vi "set_N_Dop.vi"(0 "Active":bool, 1 "Bubbler In":bool, 2 "H2 Dilute":bool, 3 "Gas Source In":bool, 4 "Run":bool, 5 "Remote":bool, 6 "Gas Flow":dbl, 8 "Flow 3":dbl, 10 "Flow 2":dbl, 12 "Flow 1":dbl) -> ()   [LabVIEW 2011]
uses:
  low_level_proc/globals.vi
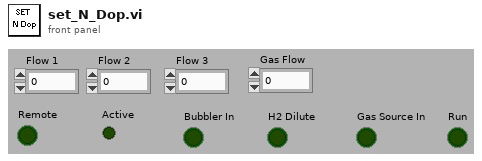
[diagram p1: front panel]
types:
  T1 = typedef "relaySpec.ctl" = cluster{"Card Index":u16, "Relay Index":u16}
  T2 = typedef "DA_Spec.ctl" = cluster{"Card Index":u16, "Channel Index":u16}
  T3 = cluster{"Relay Functions":cluster{"Remote":T1, "Active":T1, "Bubbler In":T1, "H2 dilute":T1, "Gas in":T1, "Run 2":T1}, "D/A Functions":cluster{"Flow 1":T2, "Flow 2":T2, "Flow 3":T2}, "Flow Ranges":cluster{"Flow 1 (NDOPMFC1)":u16, "Flow 2 (NDOPMFC2)":u16, "Flow 3 (NDOPMFC3)":u16, "Gas flow (NDOPMFC4)":u16}}
  T4 = cluster{"Remote":T1, "Active":T1, "Bubbler In":T1, "H2 dilute":T1, "Gas in":T1, "Run 2":T1}
  T5 = cluster{"Flow 1 (NDOPMFC1)":u16, "Flow 2 (NDOPMFC2)":u16, "Flow 3 (NDOPMFC3)":u16, "Gas flow (NDOPMFC4)":u16}
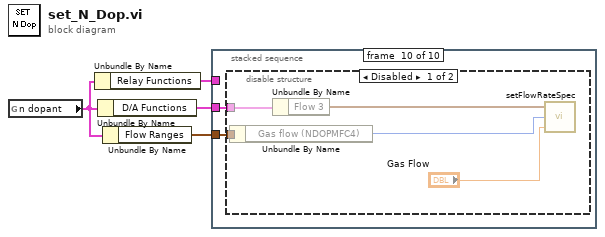
[diagram p0: block diagram]
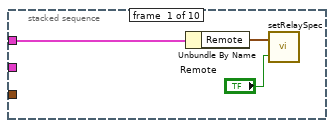
[diagram p2: hidden frame]
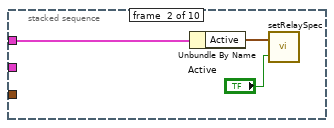
[diagram p3: hidden frame]
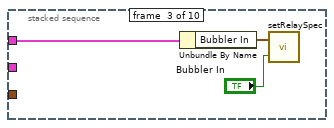
[diagram p4: hidden frame]
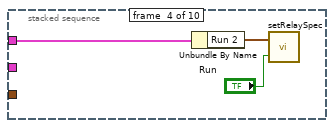
[diagram p5: hidden frame]
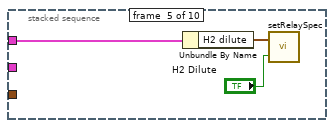
[diagram p6: hidden frame]
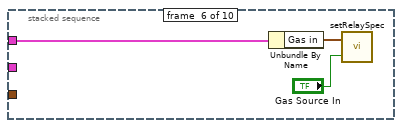
[diagram p7: hidden frame]
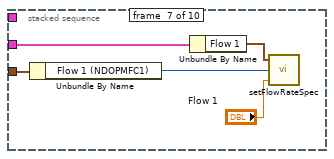
[diagram p8: hidden frame]
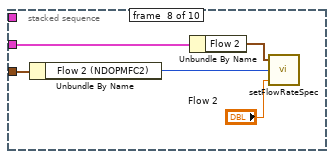
[diagram p9: hidden frame]
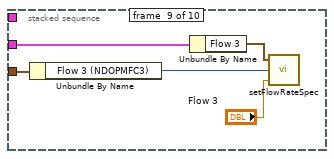
[diagram p10: hidden frame]
diagram:
  n1 = global read "globals.vi" "n dopant"() -> (w2:T3)
  n2 = Unbundle By Name(w2) -> ("Relay Functions"=w4:T4)
  n3 = Unbundle By Name(w2) -> ("D/A Functions"=w3:cluster{"Flow 1":T2, "Flow 2":T2, "Flow 3":T2})
  n4 = Unbundle By Name(w2) -> ("Flow Ranges"=w1:T5)
  n5 = stacked-sequence {
    tunnel: w4 -> [w7 w9 w12 w15 w18 w21 _ _ _ _]
    tunnel: w3 -> [_ _ _ _ _ _ w27 w31 w36 w39]
    tunnel: w1 -> [_ _ _ _ _ _ w24 w30 w35 w38]
    frame #0 {
      n6 = Unbundle By Name(w7) -> ("Remote"=w6:T1)
      n7 = call "setRelaySpec.vi"("Relay Status"="Remote", "RelaySpec"=w6) -> ()  [unwired: 1 in]
    }
    frame #1 {
      n8 = Unbundle By Name(w9) -> ("Active"=w8:T1)
      n9 = call "setRelaySpec.vi"("Relay Status"="Active", "RelaySpec"=w8) -> ()  [unwired: 1 in]
    }
    frame #2 {
      n10 = Unbundle By Name(w12) -> ("Bubbler In"=w11:T1)
      n11 = call "setRelaySpec.vi"("Relay Status"="Bubbler In", "RelaySpec"=w11) -> ()  [unwired: 1 in]
    }
    frame #3 {
      n12 = Unbundle By Name(w15) -> ("Run 2"=w14:T1)
      n13 = call "setRelaySpec.vi"("Relay Status"="Run", "RelaySpec"=w14) -> ()  [unwired: 1 in]
    }
    frame #4 {
      n14 = Unbundle By Name(w18) -> ("H2 dilute"=w17:T1)
      n15 = call "setRelaySpec.vi"("Relay Status"="H2 Dilute", "RelaySpec"=w17) -> ()  [unwired: 1 in]
    }
    frame #5 {
      n16 = Unbundle By Name(w21) -> ("Gas in"=w20:T1)
      n17 = call "setRelaySpec.vi"("Relay Status"="Gas Source In", "RelaySpec"=w20) -> ()  [unwired: 1 in]
    }
    frame #6 {
      n18 = Unbundle By Name(w24) -> ("Flow 1 (NDOPMFC1)"=w23:u16)
      n19 = Unbundle By Name(w27) -> ("Flow 1"=w26:T2)
      n20 = call "setFlowRateSpec.vi"("Flow Rate (sccm)"="Flow 1", "Flow range Index"=w23, "D/A Card"=w26) -> ()  [unwired: 2 in]
    }
    frame #7 {
      n21 = Unbundle By Name(w30) -> ("Flow 2 (NDOPMFC2)"=w29:u16)
      n22 = Unbundle By Name(w31) -> ("Flow 2"=w28:T2)
      n23 = call "setFlowRateSpec.vi"("Flow Rate (sccm)"="Flow 2", "Flow range Index"=w29, "D/A Card"=w28) -> ()  [unwired: 2 in]
    }
    frame #8 {
      n24 = Unbundle By Name(w35) -> ("Flow 3 (NDOPMFC3)"=w33:u16)
      n25 = Unbundle By Name(w36) -> ("Flow 3"=w34:T2)
      n26 = call "setFlowRateSpec.vi"("Flow Rate (sccm)"="Flow 3", "Flow range Index"=w33, "D/A Card"=w34) -> ()  [unwired: 2 in]
    }
    frame #9 {
      n27 = disable-structure shown="Disabled" {
        disable-tunnel: w39 -> [w44 _]
        disable-tunnel: w38 -> [w43 _]
        frame Disabled {
          n28 = Unbundle By Name(w43) -> ("Gas flow (NDOPMFC4)"=w41:u16)
          n29 = Unbundle By Name(w44) -> ("Flow 3"=w40:T2)
          n30 = call "setFlowRateSpec.vi"("Flow Rate (sccm)"="Gas Flow", "Flow range Index"=w41, "D/A Card"=w40) -> ()  [unwired: 2 in]
        }
        frame Enabled {
        }
      }
    }
  }
